vi "UT_Helper_Main.vi"(8 "error in":errorcluster) -> (0 "error out":errorcluster)   [LabVIEW 2016, in "UT_Helper.lvlib"]
doc: "Collection of tests of Logging Helpers."
uses:
  UT_Helper.lvlib
  <vilib>/addons/_JKI Toolkits/Caraya/classes/Test/Test.lvclass
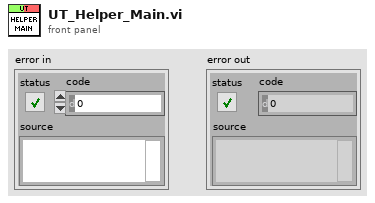
[diagram p1: front panel]
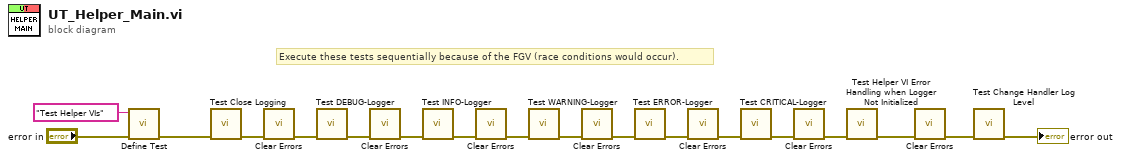
[diagram p0: block diagram]
diagram:
  # "Execute these tests sequentially because of the FGV (race conditions would occur)."
  n1 = call <vilib>:"Define Test.vi"("error in (no error)"="error in", "Label (VI Title)"="Test Helper VIs") -> ("error out"=w17:errorcluster)  [unwired: 8 in, 1 out]
  n2 = call "Test Close Logging.vi"("error in"=w17) -> ("error out"=w16:errorcluster)  [unwired: 10 in]
  n3 = call <vilib>:"Clear Errors.vi"("error in (no error)"=w16) -> ("error out"=w15:errorcluster)  [unwired: 5 in, 1 out]
  n4 = call "Test DEBUG-Logger.vi"("error in"=w15) -> ("error out"=w14:errorcluster)  [unwired: 10 in]
  n5 = call <vilib>:"Clear Errors.vi"("error in (no error)"=w14) -> ("error out"=w13:errorcluster)  [unwired: 5 in, 1 out]
  n6 = call "Test INFO-Logger.vi"("error in"=w13) -> ("error out"=w12:errorcluster)  [unwired: 10 in]
  n7 = call <vilib>:"Clear Errors.vi"("error in (no error)"=w12) -> ("error out"=w11:errorcluster)  [unwired: 5 in, 1 out]
  n8 = call "Test WARNING-Logger.vi"("error in"=w11) -> ("error out"=w10:errorcluster)  [unwired: 10 in]
  n9 = call <vilib>:"Clear Errors.vi"("error in (no error)"=w10) -> ("error out"=w9:errorcluster)  [unwired: 5 in, 1 out]
  n10 = call "Test ERROR-Logger.vi"("error in"=w9) -> ("error out"=w8:errorcluster)  [unwired: 10 in]
  n11 = call <vilib>:"Clear Errors.vi"("error in (no error)"=w8) -> ("error out"=w7:errorcluster)  [unwired: 5 in, 1 out]
  n12 = call "Test CRITICAL-Logger.vi"("error in"=w7) -> ("error out"=w6:errorcluster)  [unwired: 10 in]
  n13 = call <vilib>:"Clear Errors.vi"("error in (no error)"=w6) -> ("error out"=w5:errorcluster)  [unwired: 5 in, 1 out]
  n14 = call "Test Helper VI Error Handling when Logger Not Initialized.vi"("error in"=w5) -> ("error out"=w3:errorcluster)  [unwired: 10 in]
  n15 = call <vilib>:"Clear Errors.vi"("error in (no error)"=w3) -> ("error out"=w2:errorcluster)  [unwired: 5 in, 1 out]
  n16 = call "Test Change Handler Log Level.vi"("error in"=w2) -> ("error out"=→"error out":errorcluster)  [unwired: 10 in]
